vi "Choreo_TrajectoryDifferential_New.vi"(8 "events":T1[](array[typedef]), 9 "splits":i32[](array[numeric]), 10 "samples":T2[](array[typedef]), 11 "name":string) -> (3 "ChoreoTrajectoryDifferential":T3)   [LabVIEW 2019, in "ChoreoLib.lvlib"]
doc: "Constructs a Swerve Trajectory with the specified parameters.\n \nInputs: \n -- name - string - The name of the trajectory.\n -- samples - cluster array - The samples of the trajectory.\n -- splits - integer array - The indices of the splits in the trajectory.\n -- events - cluster array - The events in the trajectory.\n\nOutputs:\n - ChoreoTrajectory - cluster - Created trajectory stat cluster"
uses:
  TypeDef/ChoreoEventMarker.ctl
  ChoreoLib.lvlib
  TypeDef/ChoreoDifferentialSample.ctl
  TypeDef/ChoreoTrajectoryDifferential.ctl
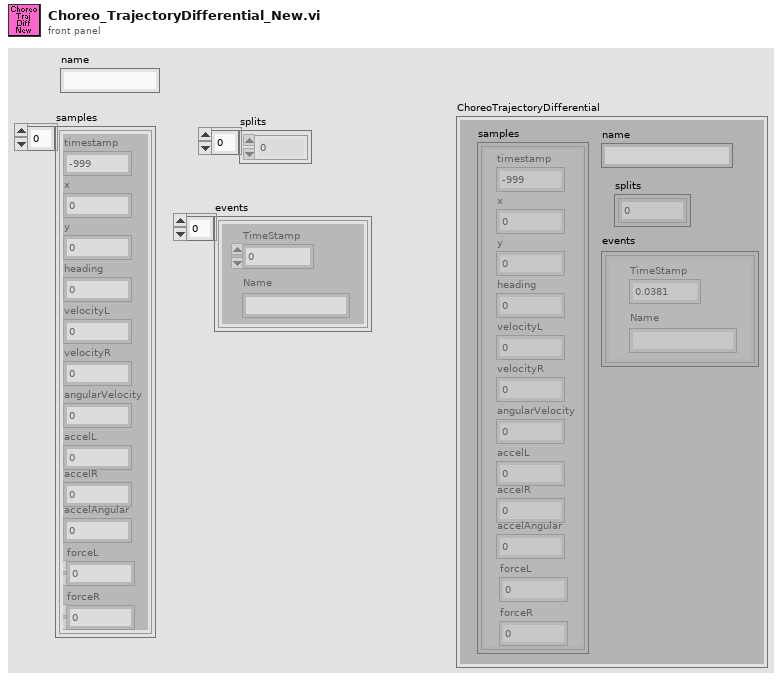
[diagram p1: front panel]
types:
  T1 = typedef "ChoreoLib.lvlib/ChoreoEventMarker.ctl" = cluster{"TimeStamp":dbl, "Name":string}
  T2 = typedef "ChoreoLib.lvlib/ChoreoDifferentialSample.ctl" = cluster{"timestamp":dbl, "x":dbl, "y":dbl, "heading":dbl, "velocityL":dbl, "velocityR":dbl, "angularVelocity":dbl, "accelL":dbl, "accelR":dbl, "accelAngular":dbl, "forceL":dbl, "forceR":dbl}
  T3 = typedef "ChoreoLib.lvlib/ChoreoTrajectoryDifferential.ctl" = cluster{"name":string, "samples":T2[], "splits":i32[], "events":T1[]}
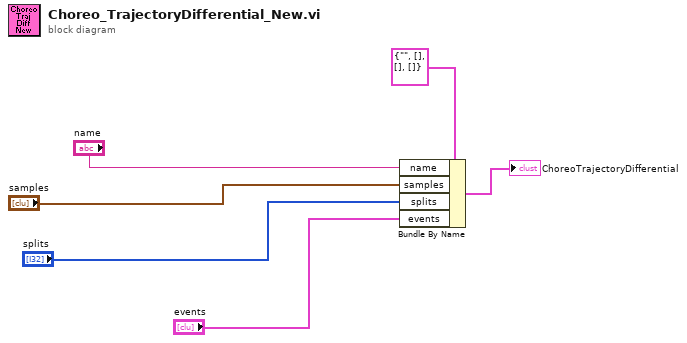
[diagram p0: block diagram]
diagram:
  n1 = Bundle By Name(cluster=T3 {"name"="", "samples"=[], "splits"=[], "events"=[]} ("ChoreoTrajectoryDifferential"), "name"="name", "samples"="samples", "splits"="splits", "events"="events") -> (→"ChoreoTrajectoryDifferential":T3)
